vi "Read.vi"(11 "State Transition Config in":refnum<class "State Transition Config.lvclass">) -> (2 "Target State":string)   [LabVIEW 2020, in "VolatusSeqConfig.lvlib" / "State Transition Config.lvclass"]
uses:
  State Transition Config.lvclass
  State Transition Config.lvclass/State Transition Config.ctl
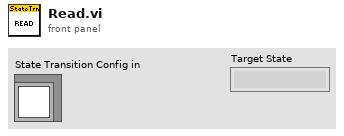
[diagram p1: front panel]
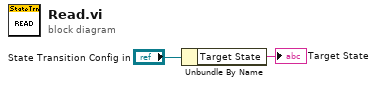
[diagram p0: block diagram]
diagram:
  n1 = Unbundle By Name("State Transition Config in") -> ("Target State"=→"Target State":string)
